vi "Increment Library Version.vi"(6 "Changes":string, 8 "error in (no error)":errorcluster, 9 "Version Increment":T2, 10 "Search Pattern":string, 11 "LabVIEW Build Script in":refnum<class "LabVIEW Build Script.lvclass">) -> (0 "error out":errorcluster, 1 "Description":string, 2 "Version":T1, 3 "LabVIEW Build Script out":refnum<class "LabVIEW Build Script.lvclass">)   [LabVIEW 2021, in "LabVIEW Build Script.lvclass"]
uses:
  LabVIEW Build Script.lvclass
  LabVIEW Build Script.lvclass/LabVIEW Build Script.ctl
  <vilib>/CIF Foundation/CIF LabVIEW Scripting/LV Scripting/LV Scripting Utilities.lvlib
  Build Script Common/Typedef/Build Script Errors.ctl
  Build Script Common/Build Script Common.lvlib
  <vilib>/CIF Foundation/CIF LabVIEW Scripting/LV Scripting/Typedef/Version Increment.ctl
  <vilib>/CIF Foundation/CIF LabVIEW Scripting/LV Scripting/Typedef/Version.ctl
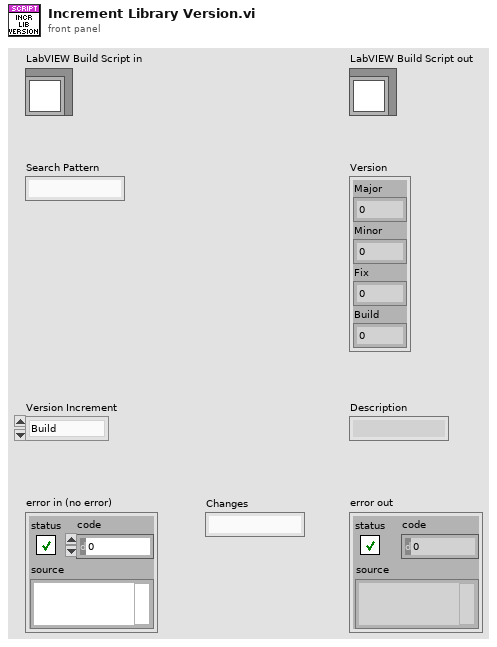
[diagram p1: front panel]
types:
  T1 = typedef "Version.ctl" = cluster{"Major":u16, "Minor":u16, "Fix":u16, "Build":u16}
  T2 = typedef "LV Scripting Utilities.lvlib/Version Increment.ctl" = enum16{"Build", "Fix", "Minor", "Major"}
  T3 = typedef "Build Script Common.lvlib/Build Script Errors.ctl" = enum16{"Item not found"}
  T4 = typedef "LV Scripting Utilities.lvlib/Library Map.ctl" = map{string, refnum<vi>}
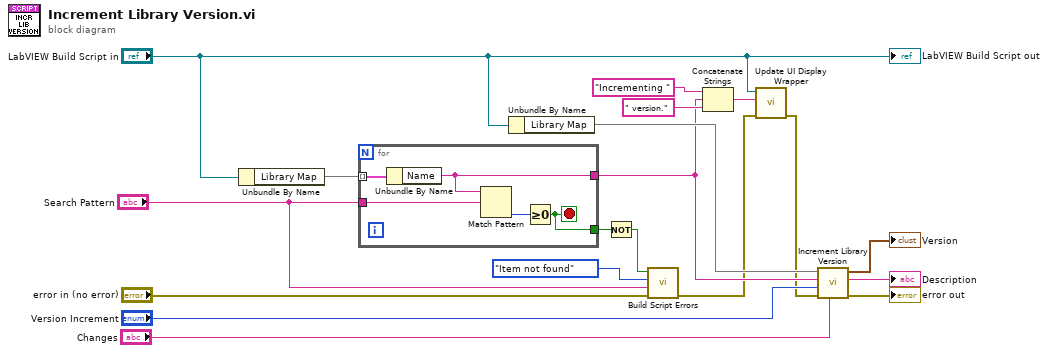
[diagram p0: block diagram]
diagram:
  n1 = Unbundle By Name("LabVIEW Build Script in") -> ("Library Map"=w16:T4)
  n2 = for {
    tunnel: w16 -> [w24] mode=indexing
    tunnel: "Search Pattern" -> [w23]
    tunnel: [w21] -> w7
    tunnel: [w20] -> w14
    stop <- w20 stop-if-true
    n3 = Unbundle By Name(w24) -> ("Name"=w21:string)
    n4 = Match Pattern(string=w21, regular expression=w23) -> (offset past match=w22:i32)  [unwired: 1 in, 3 out]
    n5 = Greater Or Equal To 0?(x=w22) -> (x >= 0?=w20:bool)
  }
  n6 = Unbundle By Name("LabVIEW Build Script in") -> ("Library Map"=w10:T4)
  n7 = Not(x=w14) -> (.not. x?=w13:bool)
  n8 = call "Build Script Errors.vi"("error in (no error)"="error in (no error)", "String to Append"="Search Pattern", "Error"=Build_Script_Errors."Item not found", "Insert Error"=w13) -> ("error out"=w5:errorcluster)  [unwired: 7 in]
  n9 = Concatenate Strings("Incrementing " ("Update for Display"), w7, " version." ("string")) -> (w18:string)
  n10 = call "Update UI Display Wrapper.vi"("error in (no error)"=w5, "Update for Display"=w18, "LabVIEW Build Script in"="LabVIEW Build Script in") -> ("error out"=w4:errorcluster)  [unwired: 8 in]
  n11 = call <vilib>:"Increment Library Version.vi"("Changes"="Changes", "error in (no error)"=w4, "Version Increment"="Version Increment", "Library Name"=w7, "Library Map"=w10) -> ("error out"=→"error out":errorcluster, "Description"=→"Description":string, "Version"=→"Version":T1)  [unwired: 4 in]
  "LabVIEW Build Script out" <- "LabVIEW Build Script in"
